vi "Write to File.vi"(8 "error in (no error)":errorcluster, 10 "header text":string, 11 "file path":path) -> (0 "error out":errorcluster)   [LabVIEW 2013, in "C Header Generator.lvlib"]
uses:
  C Header Generator.lvlib
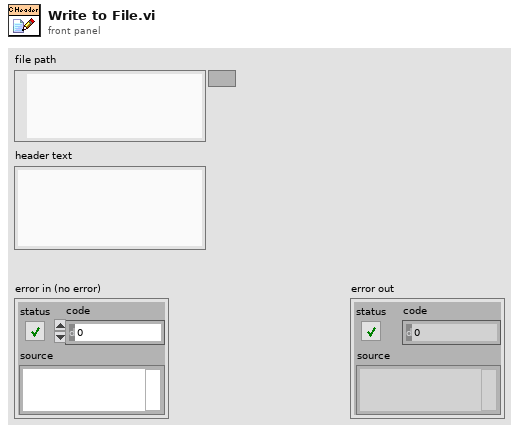
[diagram p1: front panel]
types:
  T1 = enum16{"open", "replace", "create", "open or create", "replace or create", "replace or create with confirmation"}
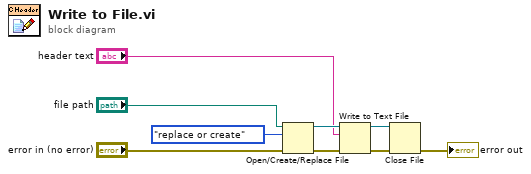
[diagram p0: block diagram]
diagram:
  n1 = Open/Create/Replace File(file path (use dialog)="file path", error in="error in (no error)", operation (0:open)=T1."replace or create") -> (refnum out=w3:refnum<file>, error out=w8:errorcluster)  [unwired: 3 in, 1 out]
  n2 = Write to Text File(file (use dialog)=w3, text="header text", error in=w8) -> (refnum out=w4:refnum<file>, error out=w7:errorcluster)  [unwired: 1 in, 1 out]
  n3 = Close File(refnum=w4, error in=w7) -> (error out=→"error out":errorcluster)  [unwired: 1 out]
